vi "4_11.vi"() -> ()   [LabVIEW 2020]
panel:
  in  "Numeric":i32
  out "Array":i32[][](array[numeric])
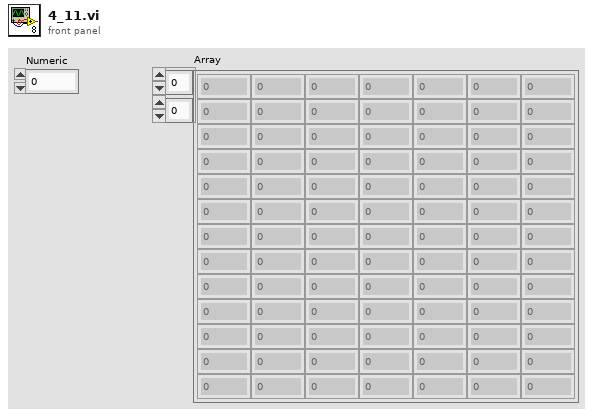
[diagram p1: front panel]
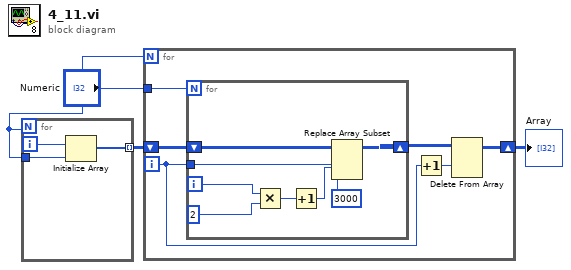
[diagram p0: block diagram]
diagram:
  n1 = for {
    N: "Numeric" -> [_]
    tunnel: "Numeric" -> [w6]
    tunnel: [w5] -> w2 mode=indexing
    i -> [w4]
    n2 = Initialize Array(w4, w6) -> (w5:i32[])
  }
  n3 = for {
    N: "Numeric" -> [_]
    shift-right: [w7] -> w3
    shift-left: w2 -> [w12]
    tunnel: "Numeric" -> [w11]
    i -> [w9]
    n4 = for {
      N: w11 -> [_]
      shift-right: [w16] -> w10
      shift-left: w12 -> [w15]
      tunnel: w9 -> [w13]
      i -> [w14]
      n5 = Multiply(x=w14, y=2) -> (x*y=w19:i32)
      n6 = Increment(x=w19) -> (x+1=w18:i32)
      n7 = Replace Array Subset(array=w15, new element=3000 ("new element/subarray"), index (row)=w13, index (col)=w18) -> (w16:i32[][])
    }
    n8 = Increment(x=w9) -> (x+1=w8:i32)
    n9 = Delete From Array(array=w10, index (row)=w8) -> (array with subset deleted=w7:i32[][])  [unwired: 2 in, 1 out]
  }
  "Array" <- w3
